vi "ComputeSampleData.vi"(10 "MeasuredVolume":dbl, 11 "UserFilledData":T2) -> (3 "MeasureData":T1)   [LabVIEW 2013]
uses:
  GlobalVariables/PreconfiguredSleeveData.vi
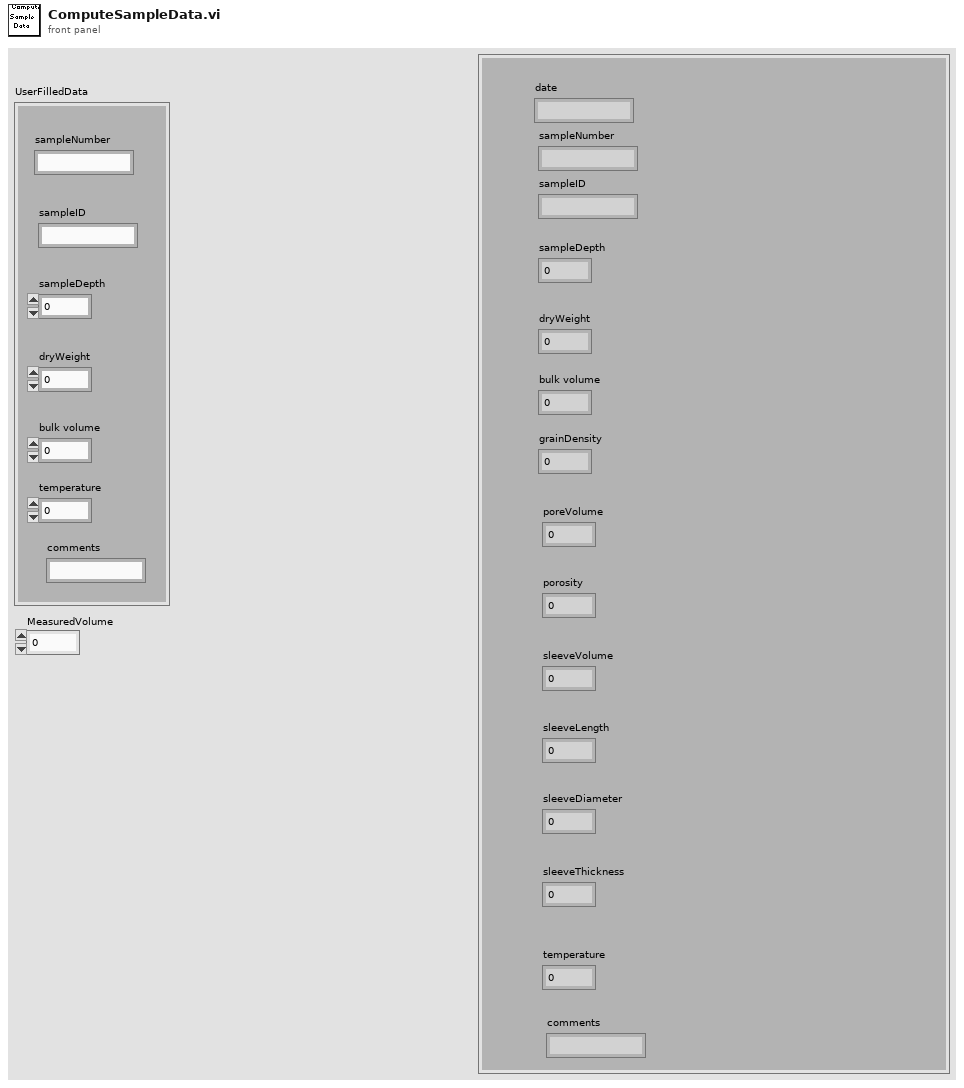
[diagram p1: front panel]
types:
  T1 = cluster{"date":string, "sampleNumber":string, "sampleID":string, "sampleDepth":dbl, "dryWeight":dbl, "grainDensity":dbl, "bulk volume":dbl, "poreVolume":dbl, "porosity":dbl, "sleeveVolume":dbl, "sleeveLength":dbl, "sleeveDiameter":dbl, "sleeveThickness":dbl, "temperature":dbl, "comments":string}
  T2 = cluster{"sampleNumber":string, "sampleID":string, "sampleDepth":dbl, "dryWeight":dbl, "bulk volume":dbl, "temperature":dbl, "comments":string}
  T3 = cluster{"sleeveLength":dbl, "sleeveDiameter":dbl, "sleeveThickness":dbl}
  T4 = cluster{string, "sampleNumber":string, "sampleID":string, "sampleDepth":dbl, "dryWeight":dbl, "bulk volume":dbl, dbl, dbl, dbl, dbl, "sleeveLength":dbl, "sleeveDiameter":dbl, "sleeveThickness":dbl, "temperature":dbl, "comments":string}
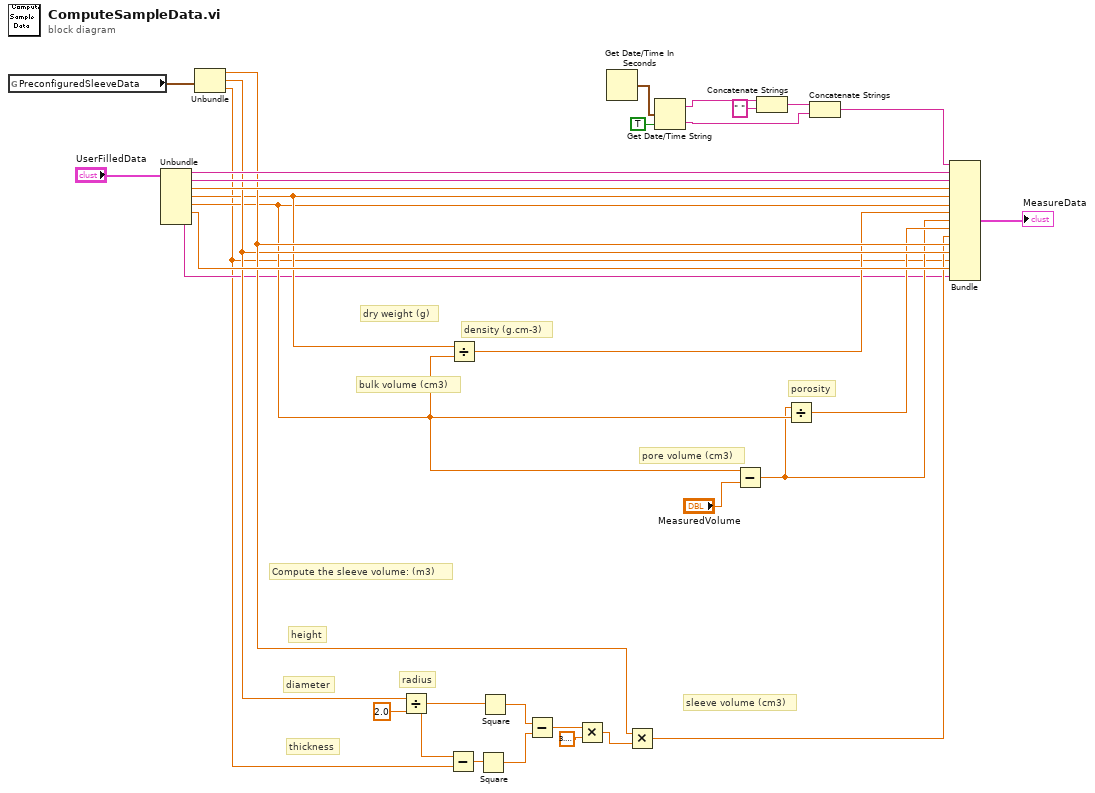
[diagram p0: block diagram]
diagram:
  # "density (g.cm-3)"
  # "porosity"
  # "sleeve volume (cm3)"
  # "pore volume (cm3)"
  # "dry weight (g)"
  # "bulk volume (cm3)"
  # "Compute the sleeve volume: (m3)"
  # "thickness"
  # "height"
  # "diameter"
  # "radius"
  n1 = global read "PreconfiguredSleeveData.vi" "PreconfiguredSleeveData"() -> (w28:T3)
  n2 = Unbundle("UserFilledData") -> ("sampleNumber"=w32:string, "sampleID"=w31:string, "sampleDepth"=w30:dbl, "dryWeight"=w16:dbl, "bulk volume"=w15:dbl, "temperature"=w29:dbl, "comments"=w10:string)
  n3 = Unbundle(w28) -> ("sleeveLength"=w18:dbl, "sleeveDiameter"=w17:dbl, "sleeveThickness"=w1:dbl)
  n4 = Divide(x=w17, y=2.0) -> (x/y=w26:dbl)
  n5 = Subtract(x=w26, y=w1) -> (x-y=w25:dbl)
  n6 = Divide(x=w16, y=w15) -> (x/y=w14:dbl)
  n7 = Square(x=w25) -> (x^2=w23:dbl)
  n8 = Square(x=w26) -> (x^2=w24:dbl)
  n9 = Subtract(x=w24, y=w23) -> (x-y=w22:dbl)
  n10 = Multiply(x=w22, y=3.141592653589793) -> (x*y=w20:dbl)
  n11 = Get Date/Time In Seconds() -> (seconds since 1Jan1904=w8:timestamp)
  n12 = Multiply(x=w18, y=w20) -> (x*y=w11:dbl)
  n13 = Get Date/Time String(seconds (now)=w8, want seconds? (F)=TRUE) -> (date string=w7:string, time string=w4:string)  [unwired: 1 in]
  n14 = Subtract(x=w15, y="MeasuredVolume") -> (x-y=w12:dbl)
  n15 = Concatenate Strings(w7, " " ("string")) -> (w5:string)
  n16 = Divide(x=w12, y=w15) -> (x/y=w13:dbl)
  n17 = Concatenate Strings(w5, w4) -> (w3:string)
  n18 = Bundle(w3, "sampleNumber"=w32, "sampleID"=w31, "sampleDepth"=w30, "dryWeight"=w16, "bulk volume"=w15, w14, w12, w13, w11, "sleeveLength"=w18, "sleeveDiameter"=w17, "sleeveThickness"=w1, "temperature"=w29, "comments"=w10) -> (→"MeasureData":T4)  [unwired: 1 in]
